vi "Alpha Calcul.vi"(10 "Coordinates 2 in":cluster{"x":i16, "y":i16}={"x"=10, "y"=10}, 11 "Coordinates 1 in":cluster{"x":i16, "y":i16}={"x"=10, "y"=10}) -> (3 "Alpha out":dbl)   [LabVIEW 2021, in "Game Board.lvclass"]
doc: "MIT Licence\nCopyright (c) 2024 David Grollier"
uses:
  Game Board.lvclass
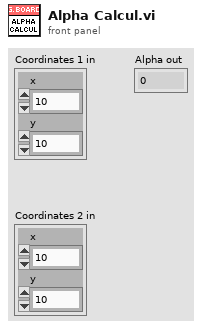
[diagram p1: front panel]
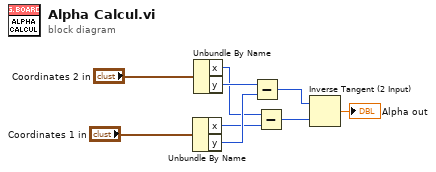
[diagram p0: block diagram]
diagram:
  n1 = Unbundle By Name("Coordinates 1 in") -> ("x"=w3:i16, "y"=w6:i16)
  n2 = Unbundle By Name("Coordinates 2 in") -> ("x"=w4:i16, "y"=w7:i16)
  n3 = Subtract(x=w7, y=w6) -> (x-y=w5:i16)
  n4 = Subtract(x=w4, y=w3) -> (x-y=w2:i16)
  n5 = Inverse Tangent (2 Input)(1:w2, 2:w5) -> (0:→"Alpha out":dbl)
